vi "UpdateHScrollbarVisibility.vi"(8 "error in (no error)":errorcluster, 11 "AdjustableMulticolumnListbox in":refnum<class "AdjMCLB.lvclass">) -> (0 "error out":errorcluster, 3 "AdjustableMulticolumnListbox out":refnum<class "AdjMCLB.lvclass">)   [LabVIEW 2020, in "AdjMCLB.lvclass"]
uses:
  AdjMCLB.lvclass
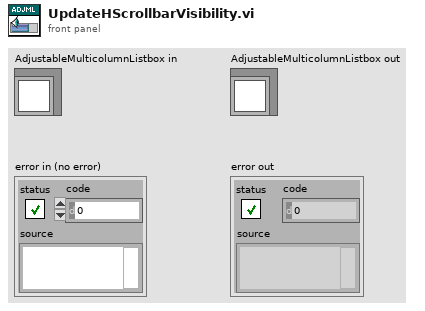
[diagram p1: front panel]
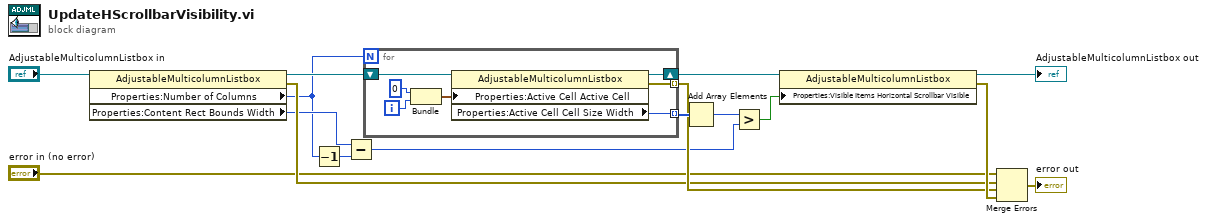
[diagram p0: block diagram]
diagram:
  n1 = property class="AdjustableMulticolumnListbox"(reference="AdjustableMulticolumnListbox in") -> (reference out=w16:refnum<class "AdjMCLB.lvclass">, error out=w10:errorcluster, "Properties:Number of Columns"=w1:u32, "Properties:Content Rect Bounds Width"=w5:i32)  [unwired: 1 in]
  n2 = Decrement(x=w1) -> (x-1=w2:u32)
  n3 = Subtract(x=w5, y=w2) -> (x-y=w3:u32)
  n4 = for {
    N: w1 -> [_]
    shift-right: [w22] -> w14
    shift-left: w16 -> [w23]
    tunnel: [w18] -> w11 mode=indexing
    tunnel: [w17] -> w15 mode=indexing
    i -> [w20]
    n5 = Bundle(0, w20) -> (w21:cluster{i32, i32})  [unwired: 1 in]
    n6 = property class="AdjustableMulticolumnListbox"(reference=w23, "Properties:Active Cell Active Cell"=w21) -> (reference out=w22:refnum<class "AdjMCLB.lvclass">, error out=w18:errorcluster, "Properties:Active Cell Cell Size Width"=w17:u32)  [unwired: 1 in]
  }
  n7 = Add Array Elements(numeric array=w15) -> (sum=w4:u32)
  n8 = Greater?(x=w4, y=w3) -> (0:w13:bool)
  n9 = property class="AdjustableMulticolumnListbox"(reference=w14, "Properties:Visible Items Horizontal Scrollbar Visible"=w13) -> (reference out=→"AdjustableMulticolumnListbox out":refnum<class "AdjMCLB.lvclass">, error out=w12:errorcluster)  [unwired: 1 in]
  n10 = Merge Errors("error in (no error)", w10, w11, w12) -> (→"error out":errorcluster)
